vi "practice7.vi"() -> ()   [LabVIEW 2018]
panel:
  in  "シャッタースピード変更":bool
  in  "選択１（画像サイズデフォルト）":bool
  in  "画像サイズ":dbl
  out "シャッター":bool
  in  "露光時間":dbl
  in  "シャッタースピード":dbl
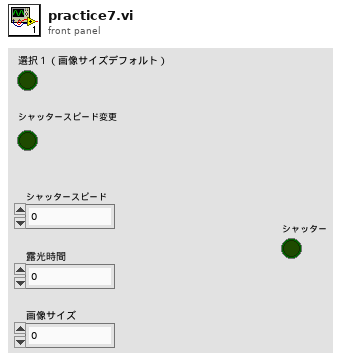
[diagram p1: front panel]
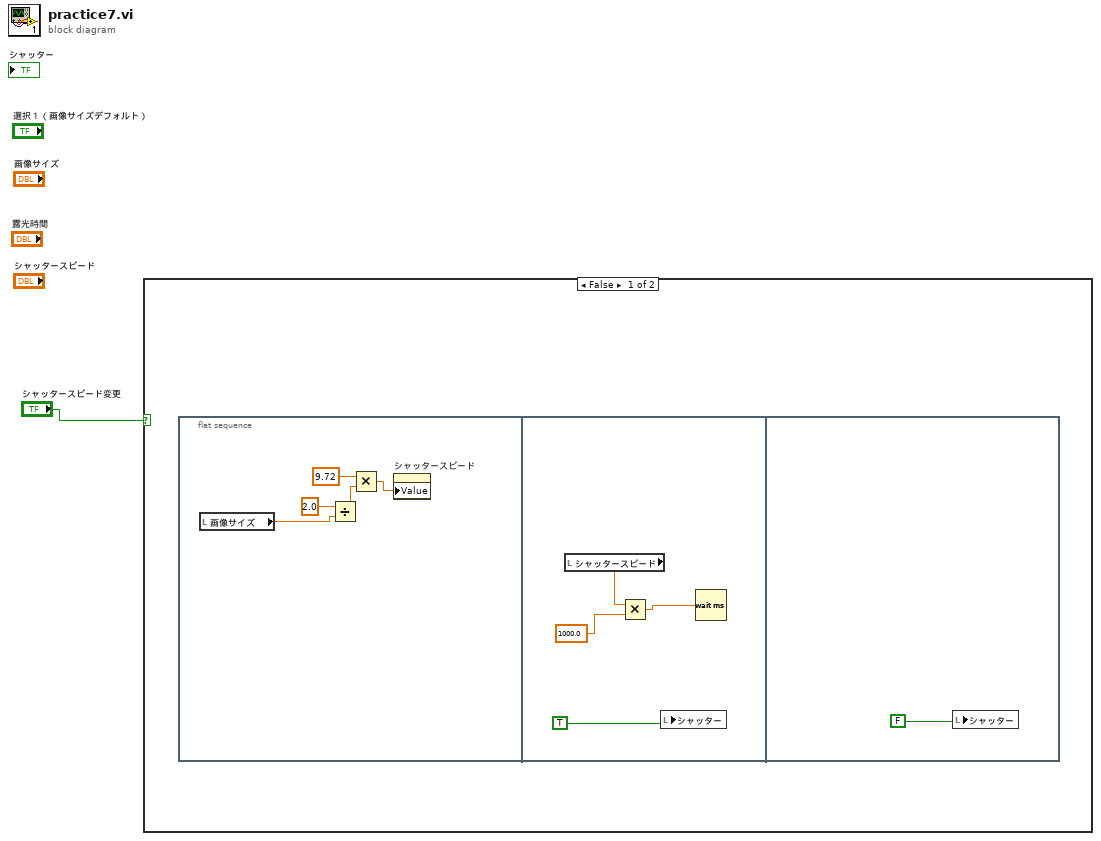
[diagram p0: block diagram]
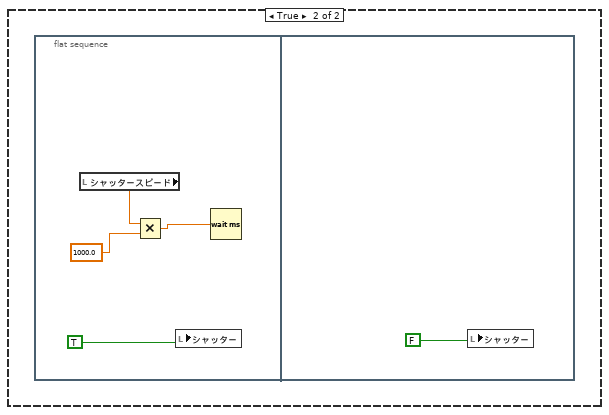
[diagram p2: hidden frame]
diagram:
  n1 = case shown="FALSE" "シャッタースピード変更" {
    frame False {
      n2 = flat-sequence {
        frame #0 {
          n3 = local read "画像サイズ"() -> (w2:dbl)
          n4 = Divide(x=2.0, y=w2) -> (x/y=w5:dbl)
          n5 = Multiply(x=9.72, y=w5) -> (x*y=w6:dbl)
          n6 = property on="シャッタースピード" class="DigNum (指定)"("Value"=w6) -> ()  [unwired: 2 in, 2 out]
        }
        frame #1 {
          n7 = local read "シャッタースピード"() -> (w7:dbl)
          n8 = Multiply(x=w7, y=1000.0 ("x*y")) -> (x*y=w8:dbl)
          n9 = local write "シャッター"(TRUE ("ブール")) -> ()
          n10 = Wait (ms)(milliseconds to wait=w8) -> ()  [unwired: 1 out]
        }
        frame #2 {
          n11 = local write "シャッター"(FALSE ("ブール")) -> ()
        }
      }
    }
    frame True {
      n12 = flat-sequence {
        frame #0 {
          n13 = local read "シャッタースピード"() -> (w12:dbl)
          n14 = Multiply(x=w12, y=1000.0 ("x*y")) -> (x*y=w13:dbl)
          n15 = local write "シャッター"(TRUE ("ブール")) -> ()
          n16 = Wait (ms)(milliseconds to wait=w13) -> ()  [unwired: 1 out]
        }
        frame #1 {
          n17 = local write "シャッター"(FALSE ("ブール")) -> ()
        }
      }
    }
  }
